vi "ReadMeasuresNode.vi"(8 "Error In":errorcluster, 11 "Keithley2602 Node In":refnum<k20>) -> (0 "Error Out":errorcluster, 2 "Measures Configuration":T1[](array[typedef]) {"Count" min=1 step=1}, 3 "Keithley2602 Node Out":refnum<k20>)   [LabVIEW 2012]
uses:
  MeasureConfiguration.ctl
  <vilib>/xml/NI_XML.lvlib
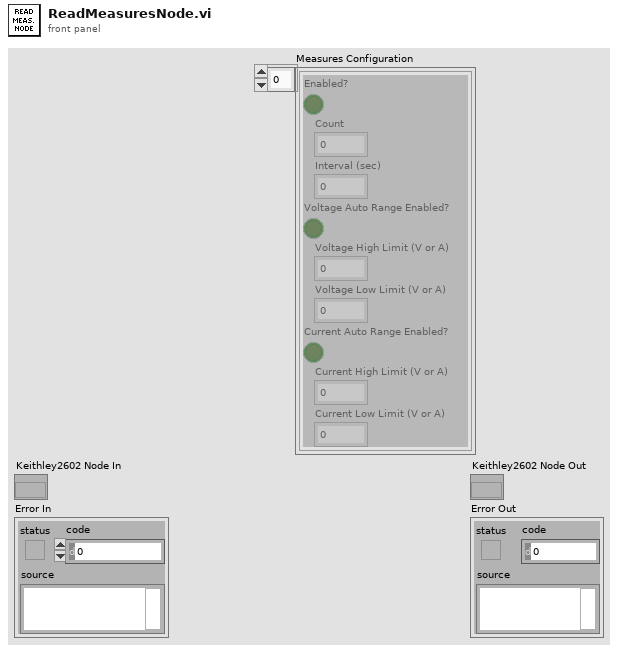
[diagram p1: front panel]
types:
  T1 = typedef "MeasureConfiguration.ctl" = cluster{"Enabled?":bool, "Count":u8, "Interval (sec)":dbl, "Voltage Auto Range Enabled?":bool, "Voltage High Limit (V or A)":dbl, "Voltage Low Limit (V or A)":dbl, "Current Auto Range Enabled?":bool, "Current High Limit (V or A)":dbl, "Current Low Limit (V or A)":dbl}
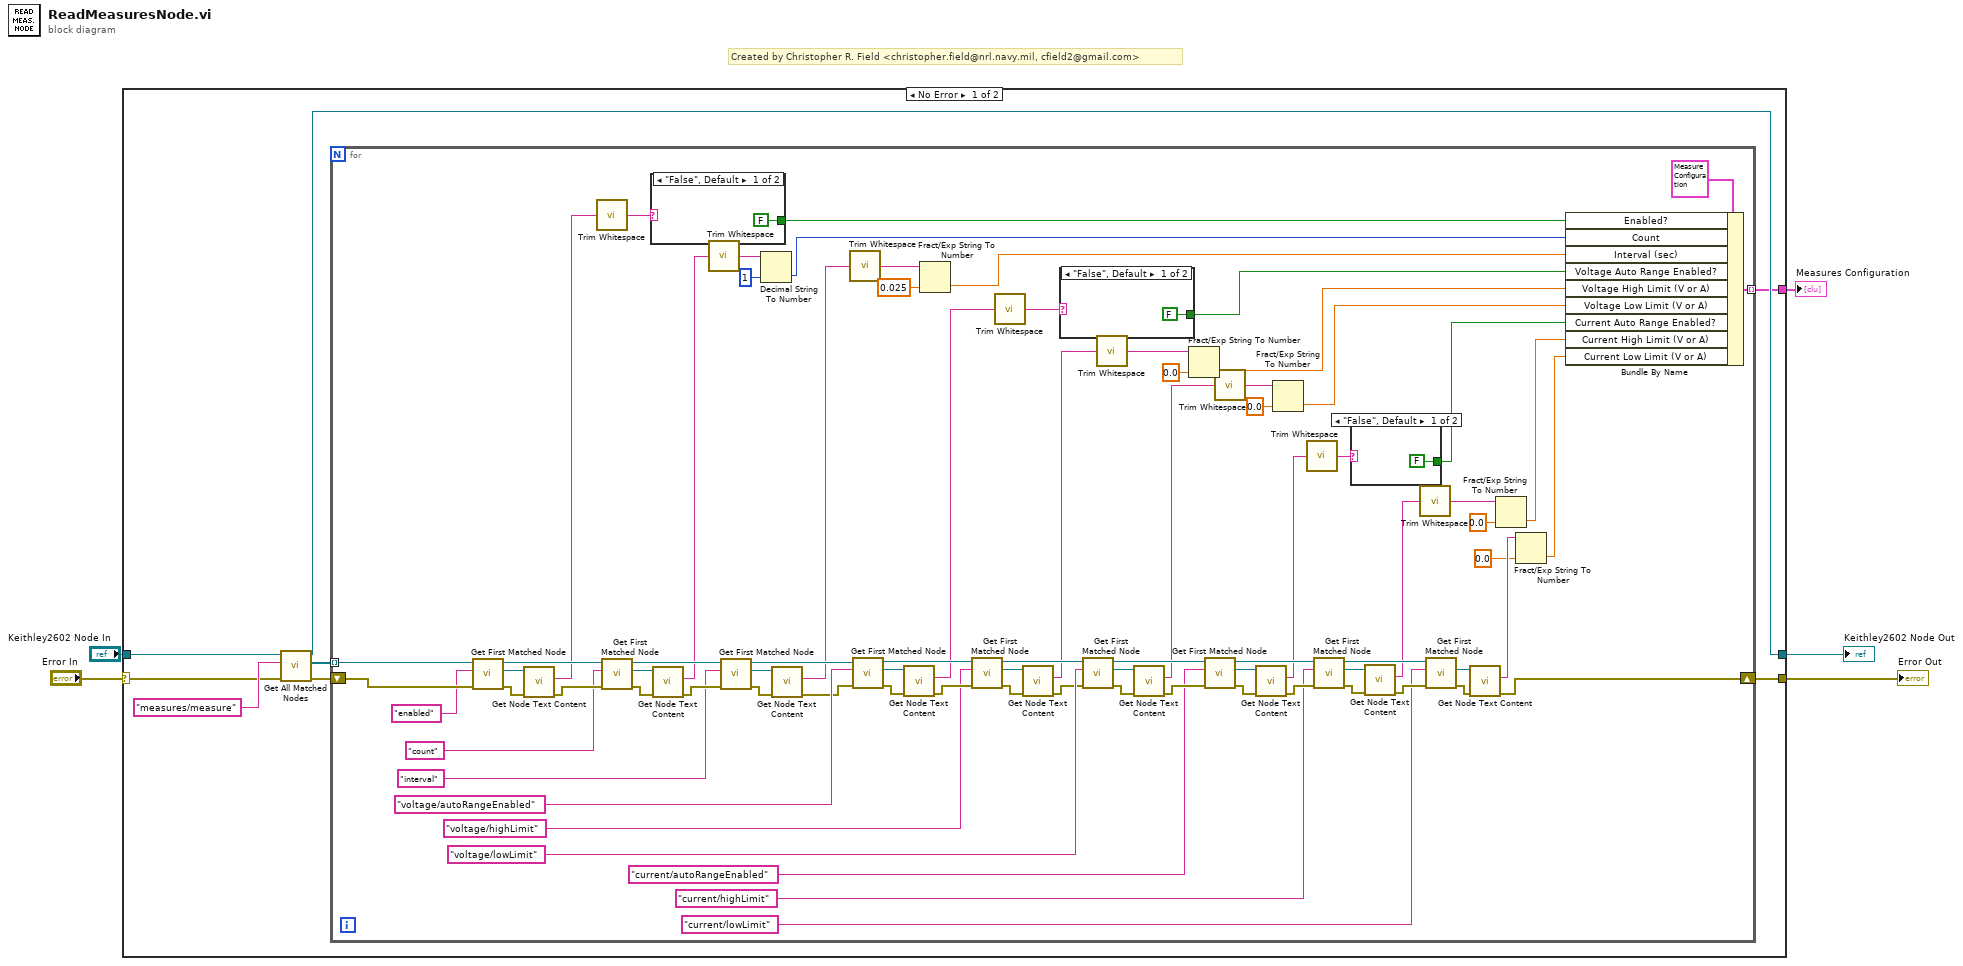
[diagram p0: block diagram]
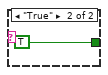
[diagram p2: hidden frame]
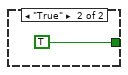
[diagram p3: hidden frame]
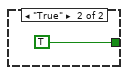
[diagram p4: hidden frame]
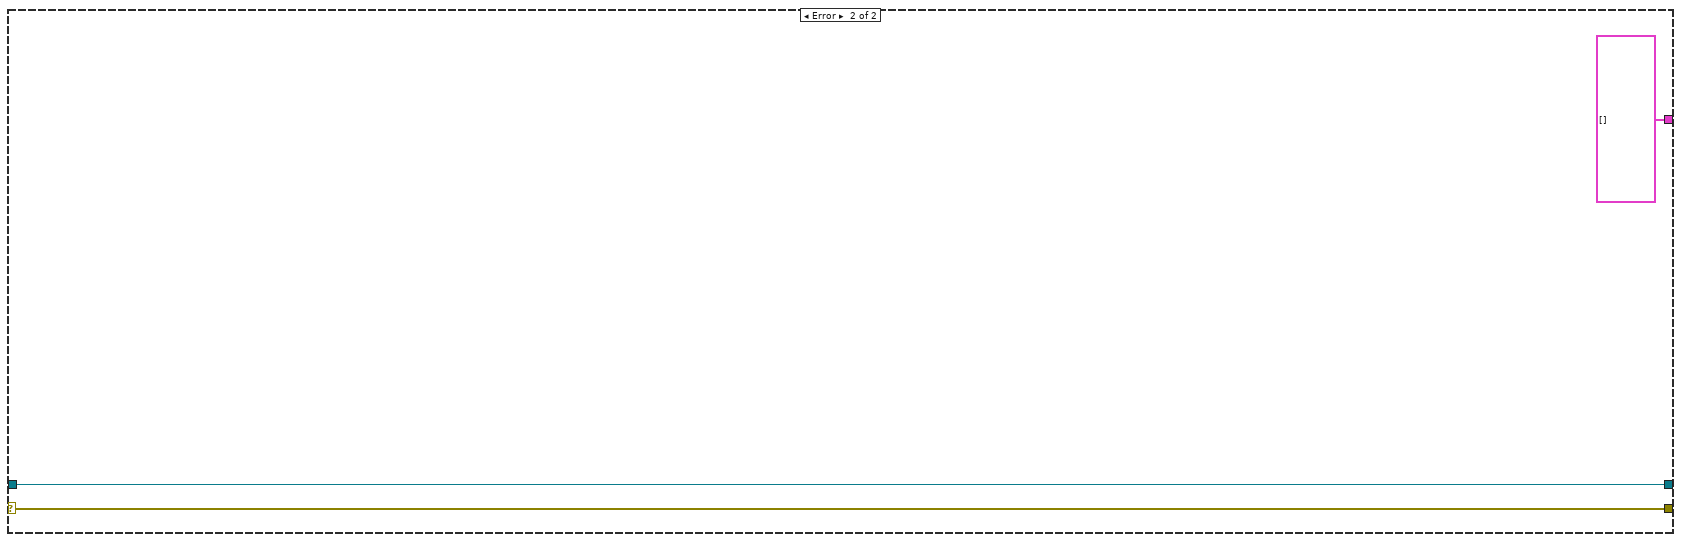
[diagram p5: hidden frame]
diagram:
  # "Created by Christopher R. Field <christopher.field@nrl.navy.mil, cfield2@gmail.com>"
  n1 = case shown="No Error" "Error In" {
    selector: "Error In" -> [w9 w101]
    tunnel: "Keithley2602 Node In" -> [w10 w102]
    tunnel: [w8 w102] -> w3
    tunnel: [w7 w101] -> w2
    tunnel: [w6 T1[] []] -> w1
    frame No Error {
      n2 = call <vilib>:"Get All Matched Nodes.vi"("error in (no error)"=w9, "XPath expression"="measures/measure", "node in"=w10) -> ("error out"=w11:errorcluster, "node result array"=w12:refnum<k20>[], "node out"=w8:refnum<k20>)  [unwired: 6 in]
      n3 = for {
        tunnel: w12 -> [w92] mode=indexing
        shift-right: [w37] -> w7
        shift-left: w11 -> [w91]
        tunnel: [w93] -> w6 mode=indexing
        n4 = call <vilib>:"Get First Matched Node.vi"("error in (no error)"=w91, "XPath expression"="enabled", "node in"=w92) -> ("error out"=w88:errorcluster, "node result"=w89:refnum<k20>, "node out"=w84:refnum<k20>)  [unwired: 6 in]
        n5 = call <vilib>:"Get Node Text Content.vi"("error in (no error)"=w88, "node in"=w89) -> ("error out"=w83:errorcluster, "node text"=w28:string)  [unwired: 7 in, 1 out]
        n6 = call <vilib>:"Trim Whitespace.vi"("string"=w28) -> ("trimmed string"=w29:string)  [unwired: 1 in]
        n7 = call <vilib>:"Get First Matched Node.vi"("error in (no error)"=w83, "XPath expression"="count", "node in"=w84) -> ("error out"=w85:errorcluster, "node result"=w86:refnum<k20>, "node out"=w79:refnum<k20>)  [unwired: 6 in]
        n8 = case shown="\"False\", Default" w29 {
          tunnel: [FALSE TRUE] -> w87
          frame "False", Default {
          }
          frame "True" {
          }
        }
        n9 = call <vilib>:"Get Node Text Content.vi"("error in (no error)"=w85, "node in"=w86) -> ("error out"=w78:errorcluster, "node text"=w26:string)  [unwired: 7 in, 1 out]
        n10 = call <vilib>:"Trim Whitespace.vi"("string"=w26) -> ("trimmed string"=w27:string)  [unwired: 1 in]
        n11 = call <vilib>:"Get First Matched Node.vi"("error in (no error)"=w78, "XPath expression"="interval", "node in"=w79) -> ("error out"=w80:errorcluster, "node result"=w81:refnum<k20>, "node out"=w72:refnum<k20>)  [unwired: 6 in]
        n12 = Decimal String To Number(string=w27, default (0L)=u32 1 ("default (0 I32)")) -> (number=w55:u32)  [unwired: 1 in, 1 out]
        n13 = call <vilib>:"Get Node Text Content.vi"("error in (no error)"=w80, "node in"=w81) -> ("error out"=w71:errorcluster, "node text"=w24:string)  [unwired: 7 in, 1 out]
        n14 = call <vilib>:"Trim Whitespace.vi"("string"=w24) -> ("trimmed string"=w25:string)  [unwired: 1 in]
        n15 = call <vilib>:"Get First Matched Node.vi"("error in (no error)"=w71, "XPath expression"="voltage/autoRangeEnabled", "node in"=w72) -> ("error out"=w74:errorcluster, "node result"=w75:refnum<k20>, "node out"=w65:refnum<k20>)  [unwired: 6 in]
        n16 = call <vilib>:"Get Node Text Content.vi"("error in (no error)"=w74, "node in"=w75) -> ("error out"=w64:errorcluster, "node text"=w22:string)  [unwired: 7 in, 1 out]
        n17 = Fract/Exp String To Number(string=w25, default (0 dbl)=0.025 ("default (0 DBL)")) -> (number=w76:dbl)  [unwired: 2 in, 1 out]
        n18 = call <vilib>:"Get First Matched Node.vi"("error in (no error)"=w64, "XPath expression"="voltage/highLimit", "node in"=w65) -> ("error out"=w68:errorcluster, "node result"=w69:refnum<k20>, "node out"=w61:refnum<k20>)  [unwired: 6 in]
        n19 = call <vilib>:"Trim Whitespace.vi"("string"=w22) -> ("trimmed string"=w23:string)  [unwired: 1 in]
        n20 = call <vilib>:"Get Node Text Content.vi"("error in (no error)"=w68, "node in"=w69) -> ("error out"=w59:errorcluster, "node text"=w20:string)  [unwired: 7 in, 1 out]
        n21 = case shown="\"False\", Default" w23 {
          tunnel: [FALSE TRUE] -> w70
          frame "False", Default {
          }
          frame "True" {
          }
        }
        n22 = call <vilib>:"Get First Matched Node.vi"("error in (no error)"=w59, "XPath expression"="voltage/lowLimit", "node in"=w61) -> ("error out"=w66:errorcluster, "node result"=w67:refnum<k20>, "node out"=w51:refnum<k20>)  [unwired: 6 in]
        n23 = call <vilib>:"Trim Whitespace.vi"("string"=w20) -> ("trimmed string"=w21:string)  [unwired: 1 in]
        n24 = call <vilib>:"Get Node Text Content.vi"("error in (no error)"=w66, "node in"=w67) -> ("error out"=w50:errorcluster, "node text"=w18:string)  [unwired: 7 in, 1 out]
        n25 = Fract/Exp String To Number(string=w21, default (0 dbl)=0.0 ("default (0 DBL)")) -> (number=w62:dbl)  [unwired: 2 in, 1 out]
        n26 = call <vilib>:"Get First Matched Node.vi"("error in (no error)"=w50, "XPath expression"="current/autoRangeEnabled", "node in"=w51) -> ("error out"=w52:errorcluster, "node result"=w53:refnum<k20>, "node out"=w48:refnum<k20>)  [unwired: 6 in]
        n27 = call <vilib>:"Trim Whitespace.vi"("string"=w18) -> ("trimmed string"=w19:string)  [unwired: 1 in]
        n28 = call <vilib>:"Get Node Text Content.vi"("error in (no error)"=w52, "node in"=w53) -> ("error out"=w47:errorcluster, "node text"=w16:string)  [unwired: 7 in, 1 out]
        n29 = Fract/Exp String To Number(string=w19, default (0 dbl)=0.0 ("default (0 DBL)")) -> (number=w58:dbl)  [unwired: 2 in, 1 out]
        n30 = call <vilib>:"Trim Whitespace.vi"("string"=w16) -> ("trimmed string"=w17:string)  [unwired: 1 in]
        n31 = call <vilib>:"Get First Matched Node.vi"("error in (no error)"=w47, "XPath expression"="current/highLimit", "node in"=w48) -> ("error out"=w45:errorcluster, "node result"=w46:refnum<k20>, "node out"=w42:refnum<k20>)  [unwired: 6 in]
        n32 = case shown="\"False\", Default" w17 {
          tunnel: [FALSE TRUE] -> w54
          frame "False", Default {
          }
          frame "True" {
          }
        }
        n33 = call <vilib>:"Get Node Text Content.vi"("error in (no error)"=w45, "node in"=w46) -> ("error out"=w41:errorcluster, "node text"=w14:string)  [unwired: 7 in, 1 out]
        n34 = call <vilib>:"Trim Whitespace.vi"("string"=w14) -> ("trimmed string"=w15:string)  [unwired: 1 in]
        n35 = call <vilib>:"Get First Matched Node.vi"("error in (no error)"=w41, "XPath expression"="current/lowLimit", "node in"=w42) -> ("error out"=w39:errorcluster, "node result"=w38:refnum<k20>)  [unwired: 6 in, 1 out]
        n36 = call <vilib>:"Get Node Text Content.vi"("error in (no error)"=w39, "node in"=w38) -> ("error out"=w37:errorcluster, "node text"=w36:string)  [unwired: 7 in, 1 out]
        n37 = Fract/Exp String To Number(string=w15, default (0 dbl)=0.0 ("default (0 DBL)")) -> (number=w43:dbl)  [unwired: 2 in, 1 out]
        n38 = Fract/Exp String To Number(string=w36, default (0 dbl)=0.0 ("default (0 DBL)")) -> (number=w35:dbl)  [unwired: 2 in, 1 out]
        n39 = Bundle By Name(cluster=T1 {"Enabled?"=FALSE, "Count"=1, "Interval (sec)"=0.025, "Voltage Auto Range Enabled?"=TRUE, "Voltage High Limit (V or A)"=0.0, "Voltage Low Limit (V or A)"=0.0, "Current Auto Range Enabled?"=TRUE, "Current High Limit (V or A)"=0.0, "Current Low Limit (V or A)"=0.0} ("Measure Configuration"), "Enabled?"=w87, "Count"=w55, "Interval (sec)"=w76, "Voltage Auto Range Enabled?"=w70, "Voltage High Limit (V or A)"=w62, "Voltage Low Limit (V or A)"=w58, "Current Auto Range Enabled?"=w54, "Current High Limit (V or A)"=w43, "Current Low Limit (V or A)"=w35) -> (w93:T1)
      }
    }
    frame Error {
    }
  }
  "Keithley2602 Node Out" <- w3
  "Error Out" <- w2
  "Measures Configuration" <- w1
